vi "_json_tmp.vi"() -> ()   [LabVIEW 2019]
uses:
  json/JSON.lvlib
panel:
  out "JSON out":string
  out "error out 2":errorcluster
  out "Keys":string[](array[string])
  out "Values":variant[](array[variant])
  out "Variant out":variant
  out "error out":errorcluster
  out "json out":string
  in  "cluster in":T1={"Boolean"=TRUE, "Integer"=-123, "Float"=3.1415, "String"="Hello World", "Array"=[1.2, 3.4, 5.6], "Null is U8 Enum"=enum."null", "Empty Object"={"Empty is U16 Enum"=enum."empty"}, "Empty Array"=[], "Nested Objects"={"Supports Path"=path "C:/Data/Test.txt", "Enums are strings"=enum."Orange"}, "Time Stamp as RFC-3339 String"=timestamp(3659220242.295989 s since 1904-01-01), "points"=[{"x"=1.0, "y"=2.0}, {"x"=3.0, "y"=4.0}]} {"Time Stamp as RFC-3339 String" format="%<%H:%M:%S%6u\n%Y/%m/%d>T"}
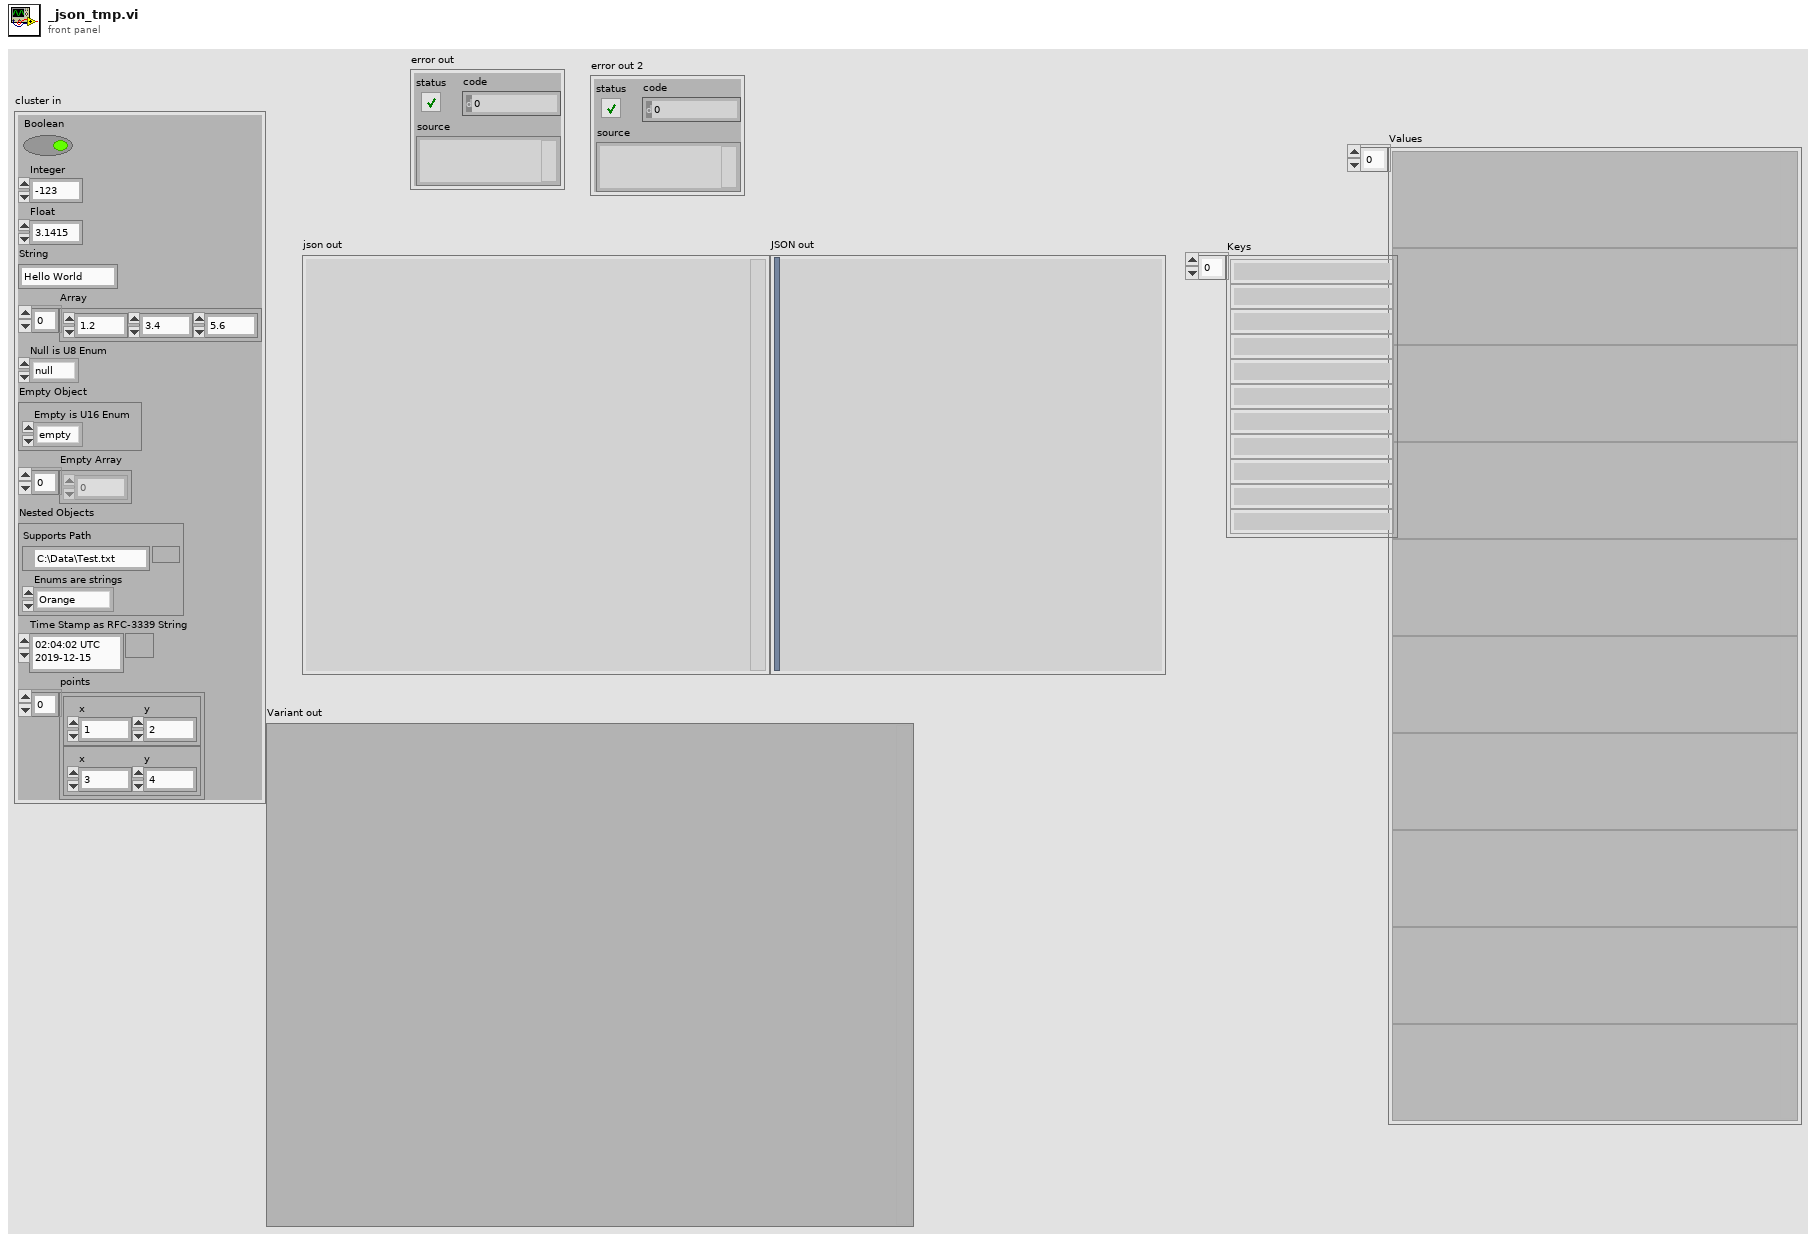
[diagram p1: front panel]
types:
  T1 = cluster{"Boolean":bool, "Integer":i32, "Float":dbl, "String":string, "Array":dbl[], "Null is U8 Enum":enum8{"null"}, "Empty Object":cluster{"Empty is U16 Enum":enum16{"empty"}}, "Empty Array":dbl[], "Nested Objects":cluster{"Supports Path":path, "Enums are strings":enum16{"Apple", "Orange", "Banana"}}, "Time Stamp as RFC-3339 String":timestamp, "points":cluster{"x":dbl, "y":dbl}[]}
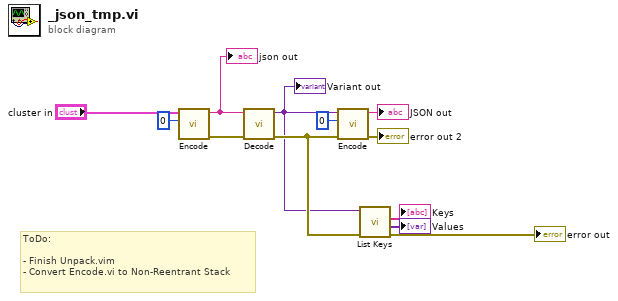
[diagram p0: block diagram]
diagram:
  # "ToDo:\n\n- Finish Unpack.vim\n- Convert Encode.vi to Non-Reentrant Stack"
  n1 = call "Encode.vi"("Pretty Indent (-1=None)"=0, "Variant in"="cluster in") -> ("error out"=w11:errorcluster, "JSON out"=w10:string)  [unwired: 8 in]
  "json out" <- w10
  n2 = call "Decode.vi"("error in (no error)"=w11, "JSON in"=w10) -> ("error out"=w5:errorcluster, "Variant out"=w4:variant)  [unwired: 8 in]
  "Variant out" <- w4
  n3 = call "Encode.vi"("error in (no error)"=w5, "Pretty Indent (-1=None)"=0, "Variant in"=w4) -> ("error out"=→"error out 2":errorcluster, "JSON out"=→"JSON out":string)  [unwired: 7 in]
  n4 = call "List Keys.vi"("error in (no error)"=w5, "Variant in"=w4) -> ("error out"=→"error out":errorcluster, "Values"=→"Values":variant[], "Keys"=→"Keys":string[])  [unwired: 6 in, 1 out]
